vi "ZigZag to I64.vi"(11 "ZigZag I64":i64) -> (3 "sint64":i64)   [LabVIEW 2020, in "LV-Proto.lvlib"]
uses:
  LV-Proto.lvlib
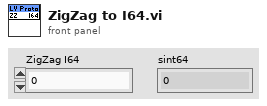
[diagram p1: front panel]
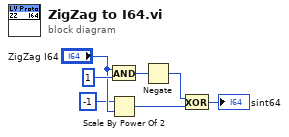
[diagram p0: block diagram]
diagram:
  n1 = And(x="ZigZag I64", y=i64 1) -> (x .and. y?=w6:i64)
  n2 = Scale By Power Of 2(n=i16 -1, x="ZigZag I64") -> (x*2^n=w3:i64)
  n3 = Negate(x=w6) -> (-x=w2:i64)
  n4 = Exclusive Or(1:w3, 2:w2) -> (0:→"sint64":i64)
